vi "getDB unique Device.vi"(8 "error in (no error)":errorcluster, 11 "Mask":string="SL066") -> (0 "error out":errorcluster, 3 "NameList":string[](array[string]))   [LabVIEW 2012]
panel:
  in  "DSN":string="DSN=behemoth-new"
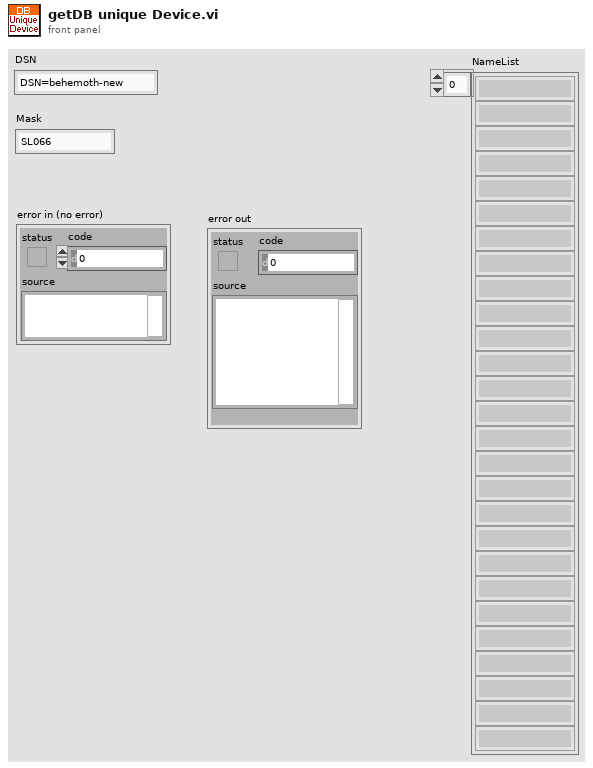
[diagram p1: front panel]
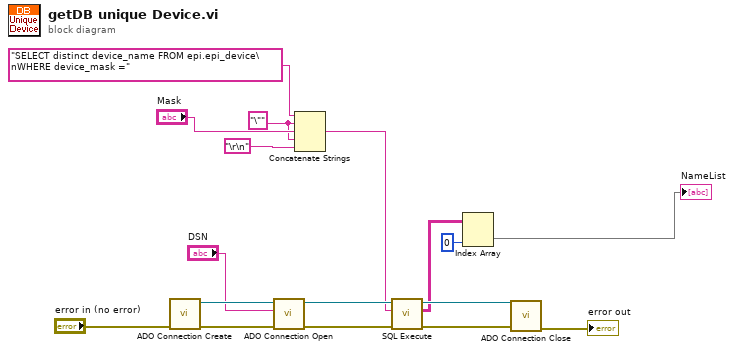
[diagram p0: block diagram]
diagram:
  w5 = "\""
  n1 = call "ADO Connection Create.vi"("error in (no error)"="error in (no error)") -> ("error out"=w15:errorcluster, "ADODB._Connection Out"=w16:refnum<k7>)  [unwired: 9 in]
  n2 = call "ADO Connection Open.vi"("error in (no error)"=w15, "ConnectionString"="DSN", "ADODB._Connection In"=w16) -> ("error out"=w12:errorcluster, "ADODB._Connection Out"=w13:refnum<k7>)  [unwired: 7 in]
  n3 = Concatenate Strings("SELECT distinct device_name FROM epi.epi_device\nWHERE device_mask =", w5, "Mask", w5, "\r\n") -> (w4:string)
  n4 = call "SQL Execute.vi"("error in (no error)"=w12, "Command Text"=w4, "ADODB._Connection In"=w13) -> ("error out"=w10:errorcluster, "Data"=w3:string[][], "ADODB._Connection Out"=w11:refnum<k7>)  [unwired: 5 in, 1 out]
  n5 = Index Array(array=w3, index (col)=0 ("disabled index (col)")) -> (element=→"NameList":string[])  [unwired: 1 in]
  n6 = call "ADO Connection Close.vi"("error in (no error)"=w10, "ADODB._Connection In"=w11) -> ("error out"=→"error out":errorcluster)  [unwired: 8 in, 1 out]
